vi "write_i.vi"(8 "error in (no error)":errorcluster, 10 "i":dbl, 11 "SpectralCoclustering in":refnum<class "SpectralCoclustering.lvclass">) -> (0 "error out":errorcluster, 3 "SpectralCoclustering out":refnum<class "SpectralCoclustering.lvclass">)   [LabVIEW 2020, in "SpectralCoclustering.lvclass"]
uses:
  SpectralCoclustering.lvclass
  SpectralCoclustering.lvclass/SpectralCoclustering.ctl
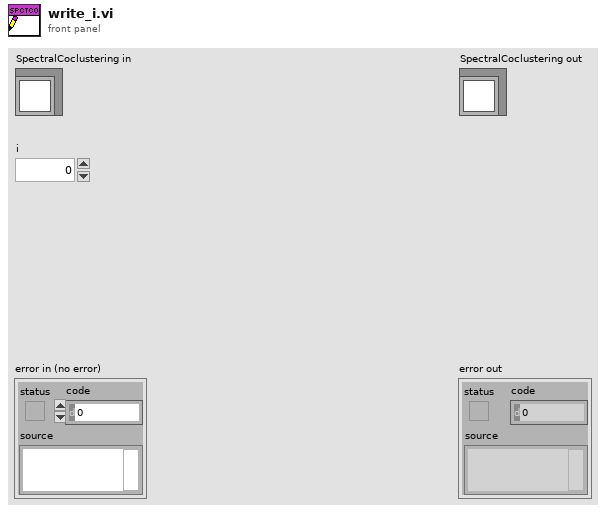
[diagram p1: front panel]
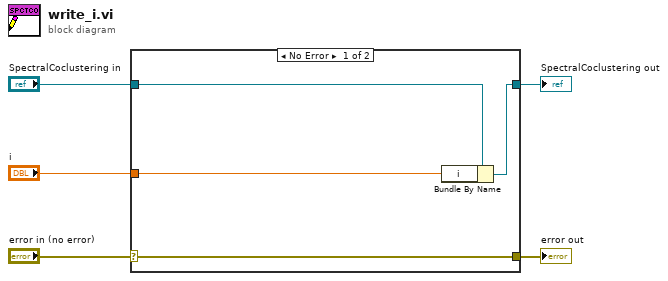
[diagram p0: block diagram]
diagram:
  n1 = case shown="No Error" "error in (no error)" {
    selector: "error in (no error)" -> [w9 w10]
    tunnel: [w9 w10] -> w4
    tunnel: [w7 w11] -> w2
    tunnel: "SpectralCoclustering in" -> [w8 w11]
    tunnel: "i" -> [w6 _]
    frame No Error {
      n2 = Bundle By Name(cluster=w8, "i"=w6) -> (w7:refnum<class "SpectralCoclustering.lvclass">)
    }
    frame Error {
    }
  }
  "error out" <- w4
  "SpectralCoclustering out" <- w2
